vi "API - PWM - Enable PWM Output.vi"(7 "Frequency":i32, 8 "error in":errorcluster, 9 "PWM Channel Number":i32, 10 "Duty Cycle (%)":i32, 11 "DAQiFi Device Properties In":T1) -> (0 "error out":errorcluster, 3 "DAQiFi Device Properties Out":T1)   [LabVIEW 2021]
doc: "Send a command to the DAQ which enables a PWM output channel, and configures frequency and duty cycle."
uses:
  TypeDefs/TypeDef - Cluster of DAQiFi Device Properties.ctl
  TypeDefs/Enum - Connection Type.ctl
  TCP - Write and Read a Synchronous Message.vi
  USB - Write and Read a Synchronous Message.vi
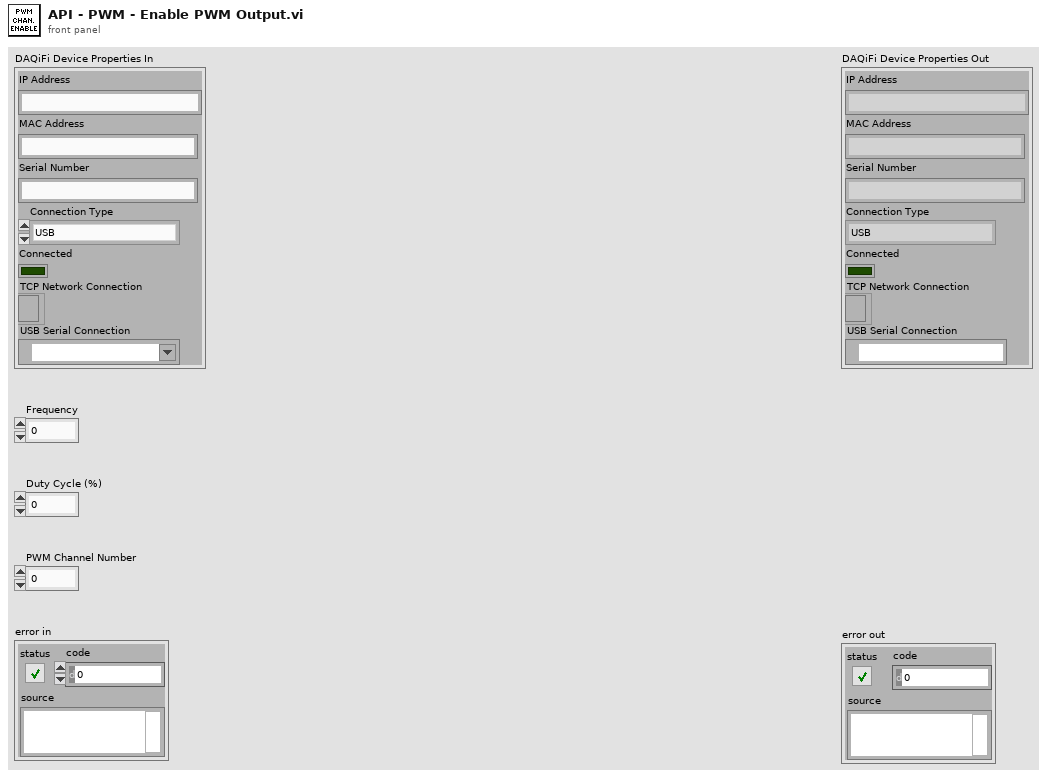
[diagram p1: front panel]
types:
  T1 = typedef "TypeDef - Cluster of DAQiFi Device Properties.ctl" = cluster{"IP Address":string, "MAC Address":string, "Serial Number":string, "Connection Type":T2, "Connected":bool, "TCP Network Connection":refnum<k5>, "USB Serial Connection":refnum<visa-resource-name>}
  T2 = typedef "Enum - Connection Type.ctl" = enum16{"USB", "TCP"}
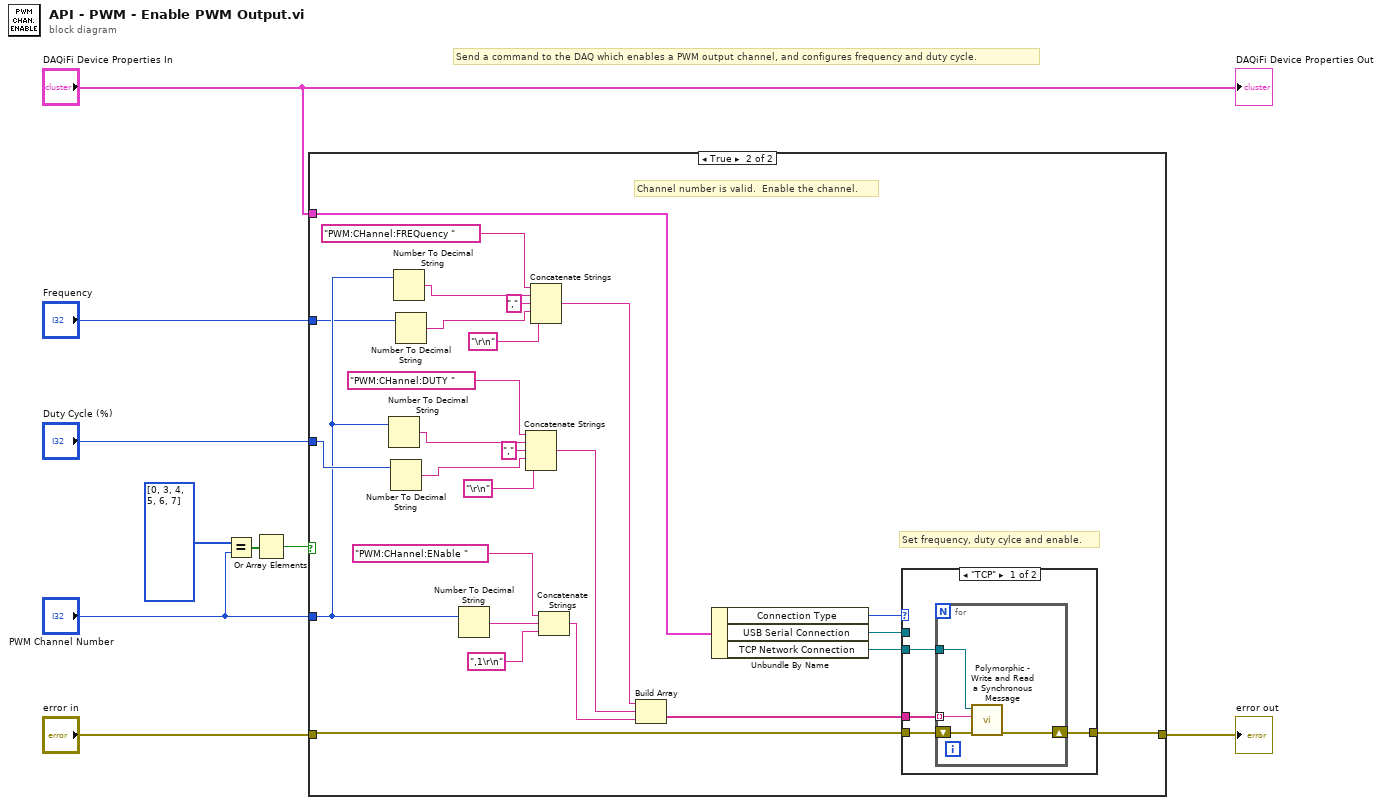
[diagram p0: block diagram]
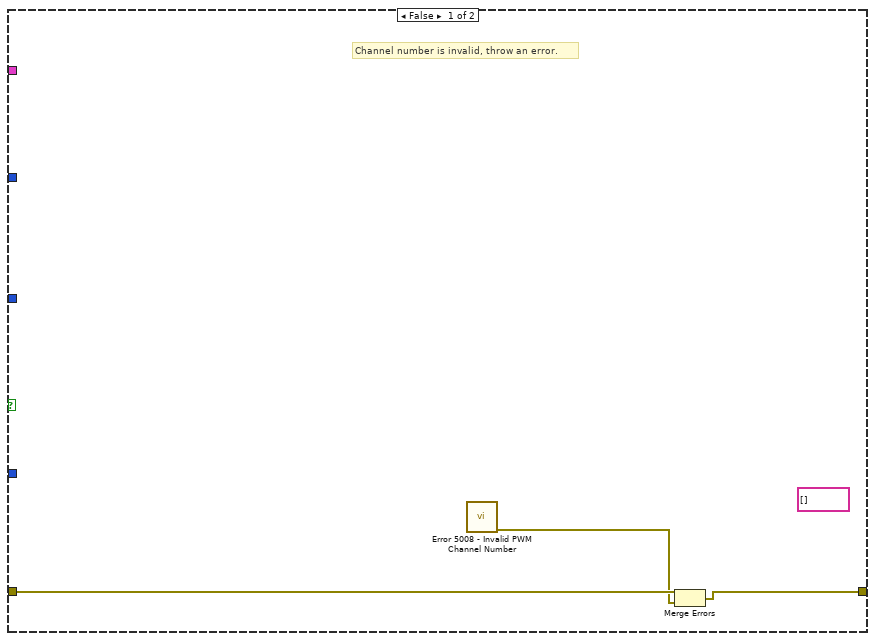
[diagram p2: hidden frame]
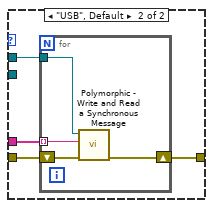
[diagram p3: hidden frame]
diagram:
  # "Send a command to the DAQ which enables a PWM output channel, and configures frequency and duty cycle."
  n1 = Equal?(x=i32[] [0, 3, 4, 5, 6, 7], y="PWM Channel Number") -> (x = y?=w4:bool[])
  n2 = Or Array Elements(Boolean array=w4) -> (logical OR=w3:bool)
  n3 = case shown="True" w3 {
    tunnel: [w11 w34] -> w9
    tunnel: "error in" -> [w12 w35]
    tunnel: "PWM Channel Number" -> [_ w18]
    tunnel: "DAQiFi Device Properties In" -> [_ w33]
    tunnel: "Duty Cycle (%)" -> [_ w28]
    tunnel: "Frequency" -> [_ w17]
    frame False {
      (unwired) string[] []
      # "Channel number is invalid, throw an error."
      n4 = call "Error 5008 - Invalid PWM Channel Number.vi"() -> ("error out"=w10:errorcluster)  [unwired: 11 in]
      n5 = Merge Errors(w12, w10) -> (w11:errorcluster)
    }
    frame True {
      # "Channel number is valid.  Enable the channel."
      # "Set frequency, duty cylce and enable."
      n6 = Number To Decimal String(number=w18) -> (decimal integer string=w27:string)  [unwired: 1 in]
      n7 = Number To Decimal String(number=w28) -> (decimal integer string=w25:string)  [unwired: 1 in]
      n8 = Number To Decimal String(number=w18) -> (decimal integer string=w22:string)  [unwired: 1 in]
      n9 = Number To Decimal String(number=w17) -> (decimal integer string=w20:string)  [unwired: 1 in]
      n10 = Number To Decimal String(number=w18) -> (decimal integer string=w37:string)  [unwired: 1 in]
      n11 = Concatenate Strings("PWM:CHannel:DUTY " ("Message to Send"), w27, "," ("string"), w25, "\r\n" ("string")) -> (w14:string)
      n12 = Concatenate Strings("PWM:CHannel:FREQuency " ("Message to Send"), w22, "," ("string"), w20, "\r\n" ("string")) -> (w15:string)
      n13 = Concatenate Strings("PWM:CHannel:ENable " ("Message to Send"), w37, ",1\r\n" ("string")) -> (w13:string)
      n14 = Build Array(w15, w14, w13) -> (w16:string[])
      n15 = Unbundle By Name(w33) -> ("Connection Type"=w32:T2, "USB Serial Connection"=w30:refnum<visa-resource-name>, "TCP Network Connection"=w31:refnum<k5>)
      n16 = case shown="\"TCP\"" w32 {
        tunnel: w35 -> [w42 w50]
        tunnel: [w41 w49] -> w34
        tunnel: w16 -> [w40 w48]
        tunnel: w31 -> [w39 _]
        tunnel: w30 -> [_ w47]
        frame "TCP" {
          n17 = for {
            tunnel: w40 -> [w44] mode=indexing
            tunnel: w39 -> [w43]
            shift-right: [w45] -> w41
            shift-left: w42 -> [w46]
            n18 = call-poly "Polymorphic - Write and Read a Synchronous Message.vi"("error in"=w46, "Message to Send"=w44, "TCP Network Connection in"=w43) -> ("error out"=w45:errorcluster)  [unwired: 6 in, 2 out]
          }
        }
        frame "USB", Default {
          n19 = for {
            tunnel: w48 -> [w52] mode=indexing
            tunnel: w47 -> [w51]
            shift-right: [w53] -> w49
            shift-left: w50 -> [w54]
            n20 = call-poly "Polymorphic - Write and Read a Synchronous Message.vi"("error in"=w54, "Message to Send"=w52, "VISA resource name in"=w51) -> ("error out"=w53:errorcluster)  [unwired: 6 in, 2 out]
          }
        }
      }
    }
  }
  "error out" <- w9
  "DAQiFi Device Properties Out" <- "DAQiFi Device Properties In"
